vi "003generate_signal_save.vi"() -> ()   [LabVIEW 2012]
uses:
  <vilib>/Utility/file.llb/Write To Spreadsheet File (DBL).vi
  <vilib>/measure/NI_MABase.lvlib
panel:
  in  "备注 2":string="原因：事件结构触发快于顺序结构，类似于中断，按下按钮时，就会保存。\n解决方案：由于顺序结构外的for循环，无法判断实际执行的位置。因此，只有放弃while循环或者放弃即开即用，即每次只能记录下一个文件或者运行前将程序面板中部分内容改为禁止，部分改为允许使用"
  in  "停止":bool
  in  "备注":string="请在运行前，选择好下面三种类型之一保存，运行时先关掉所选用的类型，接着再开启，生成的文件中请选择时间离你最远的时间查看，生成的第二个文件更改后缀名成你所需要保存的类型即可查看"
  in  "电子表格":bool
  in  "文本":bool
  in  "二进制":bool
  in  "signal type":T1(ring)
  in  "phase":dbl
  in  "amplitude":dbl=1.0
  in  "frequency":dbl=10.0
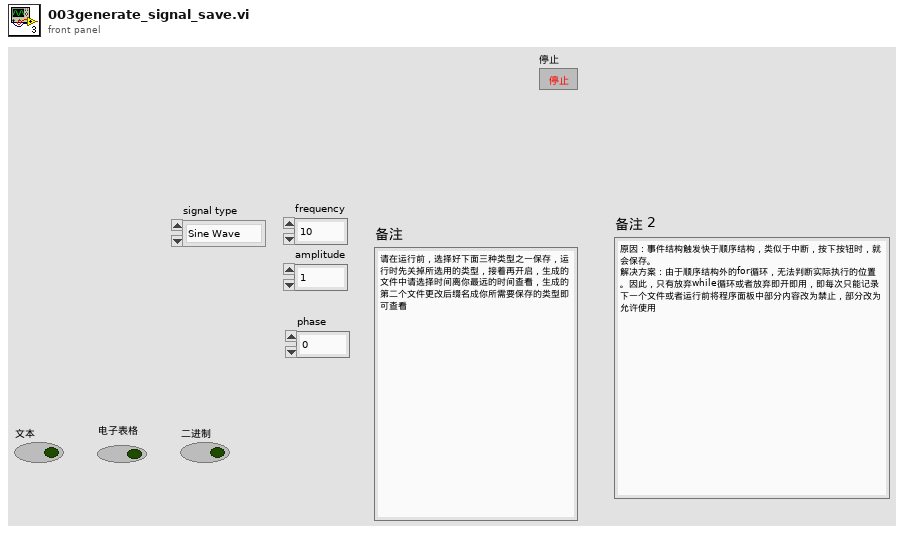
[diagram p1: front panel]
types:
  T1 = enum16{"Sine Wave", "Triangle Wave", "Square Wave", "Sawtooth Wave"}
  T2 = enum16{"open", "replace", "create", "open or create", "replace or create", "replace or create with confirmation"}
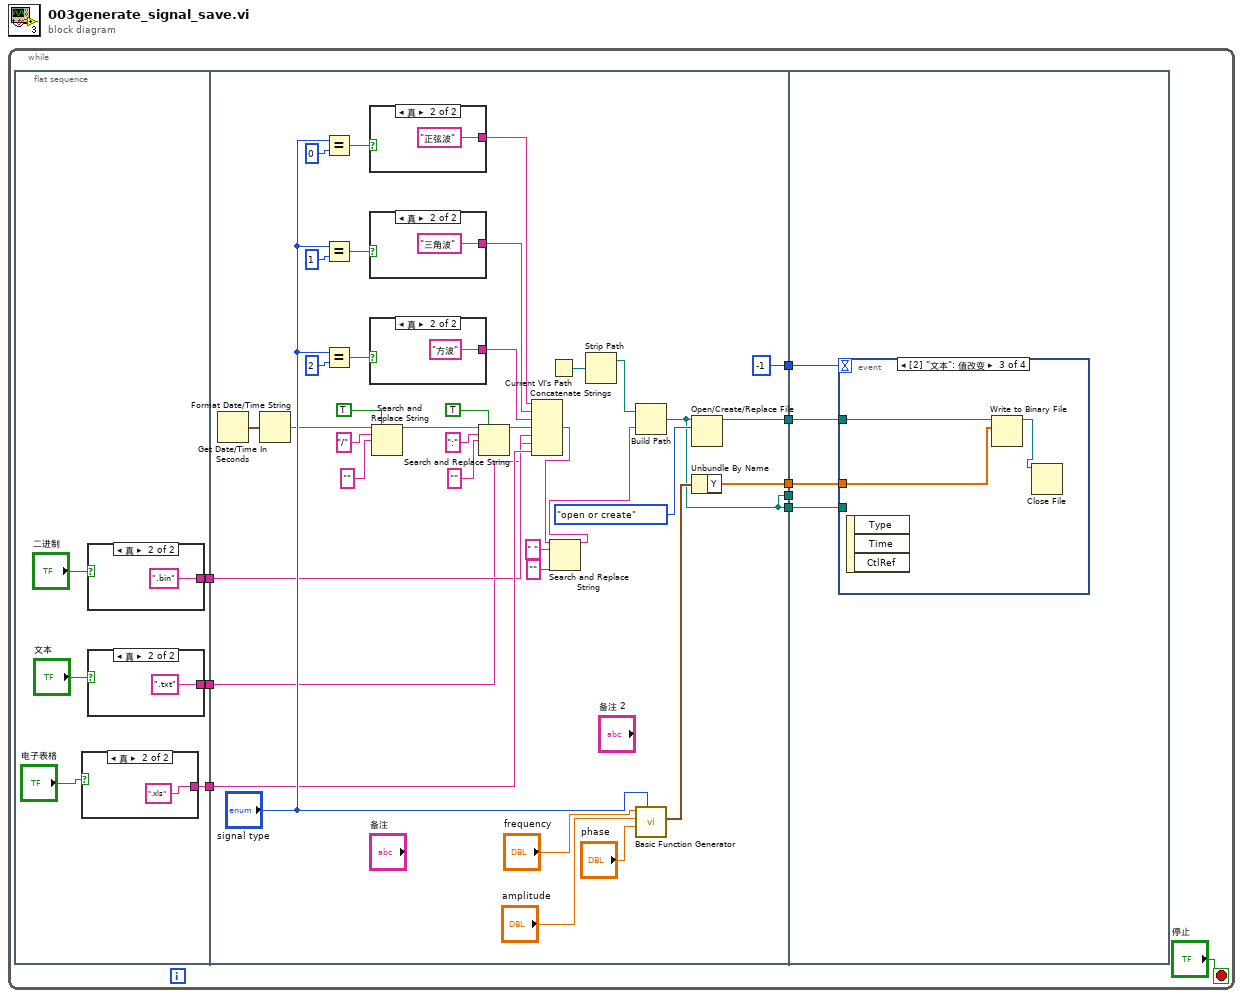
[diagram p0: block diagram]
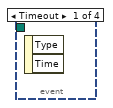
[diagram p8: hidden frame]
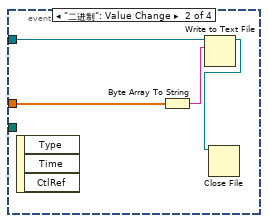
[diagram p9: hidden frame]
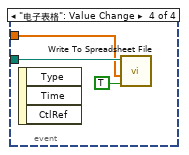
[diagram p10: hidden frame]
diagram:
  n1 = while {
    stop <- "停止" stop-if-true
    n2 = flat-sequence {
      tunnel: [w12] -> w3
      tunnel: [w11] -> w2
      tunnel: [w10] -> w1
      tunnel: [-1] -> w9
      tunnel: [w40] -> w8
      tunnel: [w26] -> w7
      tunnel: [w27] -> w6
      tunnel: [w26] -> w5
      tunnel: w3 -> [w21]
      tunnel: w2 -> [w20]
      tunnel: w1 -> [w19]
      tunnel: w5 -> [w63]
      tunnel: w6 -> [w60]
      tunnel: w7 -> [_]
      tunnel: w8 -> [w62]
      tunnel: w9 -> [w61]
      frame #0 {
        n3 = case shown="真" "电子表格" {
          tunnel: [_ ".xls" ("字符串 3")] -> w12
          frame False {
          }
          frame True {
          }
        }
        n4 = case shown="真" "二进制" {
          tunnel: [_ ".bin" ("字符串")] -> w11
          frame False {
          }
          frame True {
          }
        }
        n5 = case shown="真" "文本" {
          tunnel: [_ ".txt" ("字符串 3")] -> w10
          frame False {
          }
          frame True {
          }
        }
      }
      frame #1 {
        n6 = Get Date/Time In Seconds() -> (seconds since 1Jan1904=w37:timestamp)
        n7 = Format Date/Time String(seconds (now)=w37) -> (date/time string=w36:string)  [unwired: 2 in]
        n8 = Equal?(x="signal type", y=0) -> (x = y?=w52:bool)
        n9 = Equal?(x="signal type", y=1) -> (x = y?=w50:bool)
        n10 = Equal?(x="signal type", y=2) -> (x = y?=w48:bool)
        n11 = case shown="真" w52 {
          tunnel: [_ "正弦波" ("字符串")] -> w38
          frame False {
          }
          frame True {
          }
        }
        n12 = case shown="真" w50 {
          tunnel: [_ "三角波" ("字符串 2")] -> w39
          frame False {
          }
          frame True {
          }
        }
        n13 = case shown="真" w48 {
          tunnel: [_ "方波" ("字符串 3")] -> w43
          frame False {
          }
          frame True {
          }
        }
        n14 = Search and Replace String(replace all?=TRUE ("替换全部？(F)"), input string=w36, search string="/", replace string="") -> (result string=w32:string)  [unwired: 4 in, 3 out]
        n15 = Search and Replace String(replace all?=TRUE ("替换全部？(F)"), input string=w32, search string=":", replace string="") -> (result string=w29:string)  [unwired: 4 in, 3 out]
        n16 = Concatenate Strings(w38, w39, w43, w29, w20, w19, w21) -> (w25:string)
        n17 = Current VI's Path() -> (path=w42:path)
        n18 = Search and Replace String(input string=w25, search string=" " ("搜索字符串"), replace string="" ("替换字符串(\"\")")) -> (result string=w22:string)  [unwired: 5 in, 3 out]
        n19 = Strip Path(path=w42) -> (stripped path=w41:path)  [unwired: 1 out]
        n20 = Build Path(base path=w41, name or relative path=w22) -> (appended path=w26:path)
        n21 = call <vilib>:"Basic Function Generator.vi"("signal type"="signal type", "phase"="phase", "amplitude"="amplitude", "frequency"="frequency") -> ("signal out"=w45:waveform(dbl))  [unwired: 5 in, 2 out]
        n22 = Open/Create/Replace File(file path (use dialog)=w26, operation (0:open)=T2."open or create" ("操作(0:open)")) -> (refnum out=w40:refnum<file>)  [unwired: 4 in, 2 out]
        n23 = Unbundle By Name(w45) -> ("Y"=w27:dbl[])
      }
      frame #2 {
        n24 = event shown="[2] \"文本\": 值改变" {
          selector: _ -> [_ _ _ _]
          dyn-events: _ -> [_ _ _ _]
          timeout: w61 -> [_ _ _ _]
          tunnel: w62 -> [_ w66 w70 _]
          tunnel: w60 -> [_ w65 w69 w71]
          tunnel: w63 -> [_ _ _ w72]
          event Timeout {
            n25 = event-data() -> ()  [unwired: 1 in, 2 out]
          }
          event "二进制": Value Change {
            n26 = event-data() -> ()  [unwired: 1 in, 3 out]
            n27 = Byte Array To String(unsigned byte array=w65) -> (string=w67:string)
            n28 = Write to Text File(file (use dialog)=w66, text=w67) -> (refnum out=w64:refnum<file>)  [unwired: 2 in, 2 out]
            n29 = Close File(refnum=w64) -> ()  [unwired: 1 in, 2 out]
          }
          event "文本": Value Change {
            n30 = event-data() -> ()  [unwired: 1 in, 3 out]
            n31 = Write to Binary File(file (use dialog)=w70, data=w69) -> (refnum out=w68:refnum<file>)  [unwired: 4 in, 2 out]
            n32 = Close File(refnum=w68) -> ()  [unwired: 1 in, 2 out]
          }
          event "电子表格": Value Change {
            n33 = event-data() -> ()  [unwired: 1 in, 3 out]
            n34 = call-poly <vilib>:"Write To Spreadsheet File.vi"("append to file? (new file:F)"=TRUE, "1D data"=w71, "file path (dialog if empty)"=w72) -> ()  [unwired: 5 in, 1 out]
          }
        }
      }
    }
  }
